vi "Panel.vi"(8 "error in (no error)":errorcluster, 11 "Panel in":refnum<class "Panel.lvclass">) -> ()   [LabVIEW 2018, in "OOPanel.lvlib" / "Panel.lvclass"]
uses:
  Panel.lvclass
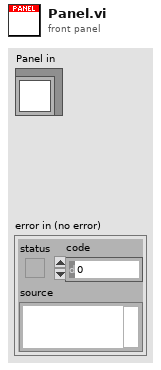
[diagram p1: front panel]
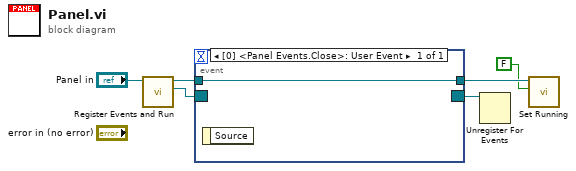
[diagram p0: block diagram]
diagram:
  n1 = call "Register Events and Run.vi"("Panel in"="Panel in") -> ("Event Registration Refnum"=w5:refnum<event-registration>, "Panel out"=w4:refnum<class "Panel.lvclass">)  [unwired: 8 in, 1 out]
  n2 = event shown="[0] <Panel Events.Close>: User Event" {
    selector: w5 -> [_]
    dyn-events: [_] -> w1
    timeout: _ -> [_]
    tunnel: w4 -> [w7]
    tunnel: [w7] -> w3
    event User Event {
      n3 = event-data() -> ()  [unwired: 1 in, 1 out]
    }
  }
  n4 = Unregister For Events(event registration refnum=w1) -> ()  [unwired: 1 in, 1 out]
  n5 = call "Set Running.vi"("Running"=FALSE, "Panel in"=w3) -> ()  [unwired: 8 in, 2 out]
